vi "Initialise.vi"(11 "Size":u16 format="%04x") -> (3 "EEPROM out":refnum<class "EEPROM.lvclass">)   [LabVIEW 2021, in "EEPROM.lvclass"]
uses:
  EEPROM.lvclass
  EEPROM.lvclass/EEPROM.ctl
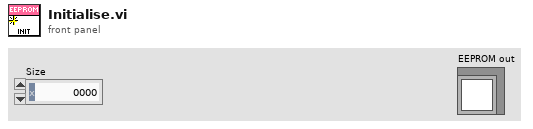
[diagram p1: front panel]
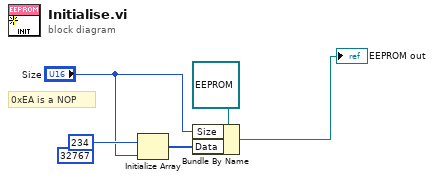
[diagram p0: block diagram]
diagram:
  (unwired) 32767 ("dimension size")
  # "0xEA is a NOP"
  n1 = Initialize Array(u8 234 ("element"), "Size") -> (w3:u8[])
  n2 = Bundle By Name(cluster=refnum<class "EEPROM.lvclass"> refnum ("EEPROM in"), "Size"="Size", "Data"=w3) -> (→"EEPROM out":refnum<class "EEPROM.lvclass">)
